vi "calc target data.vi"(8 "error in (no error)":errorcluster) -> (0 "error out":errorcluster, 1 "D":dbl=167.6323165634755, 2 "TARGET (XY)":T1 {"Y" format="%.4g"; "X" format="%.4g"}, 3 "steer (deg)":dbl=-10.0)   [LabVIEW 2023]
uses:
  ctrl defs/ctrl XY coord.ctl
  Global odometry.vi
  Global INIT.vi
  <vilib>/Rock Robotics/WPI/ThirdParty/JAS_Junk/TrajLib/Trajectory_Library.lvlib
panel:
  out "Inches":dbl
  out "DistanceToTarget_Meters":dbl
  in  "TEST":bool
  out "Dx":dbl=-165.57299375482046
  out "Dy":dbl=26.19498607564902
  out "ty":dbl=-15.0
  out "tx":dbl=-10.0
  out "tx angle error":dbl
  out "angle":dbl=22.0
  out "Z":dbl=22.0
  out "Y":dbl=-3.0
  out "X":dbl
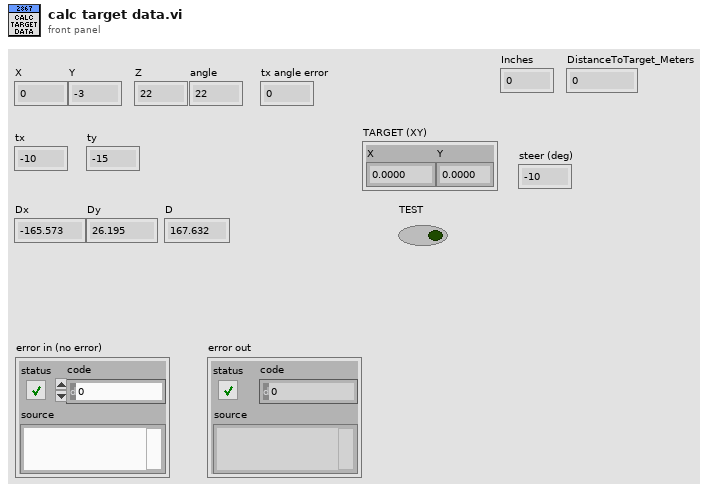
[diagram p1: front panel]
types:
  T1 = typedef "ctrl XY coord.ctl" = cluster{"X":dbl, "Y":dbl}
  T2 = typedef "ctrl LIMELIGHT initialize.ctl" = cluster{"Installed?":bool, "pose":cluster{"X":dbl, "Y":dbl, "Z":dbl, "angle to horizon":dbl, "tx angle offset":dbl}}
  T3 = typedef "ctrl LimeLight target.ctl" = cluster{"tv":u8, "tx":dbl, "ty":dbl, "ta":dbl}
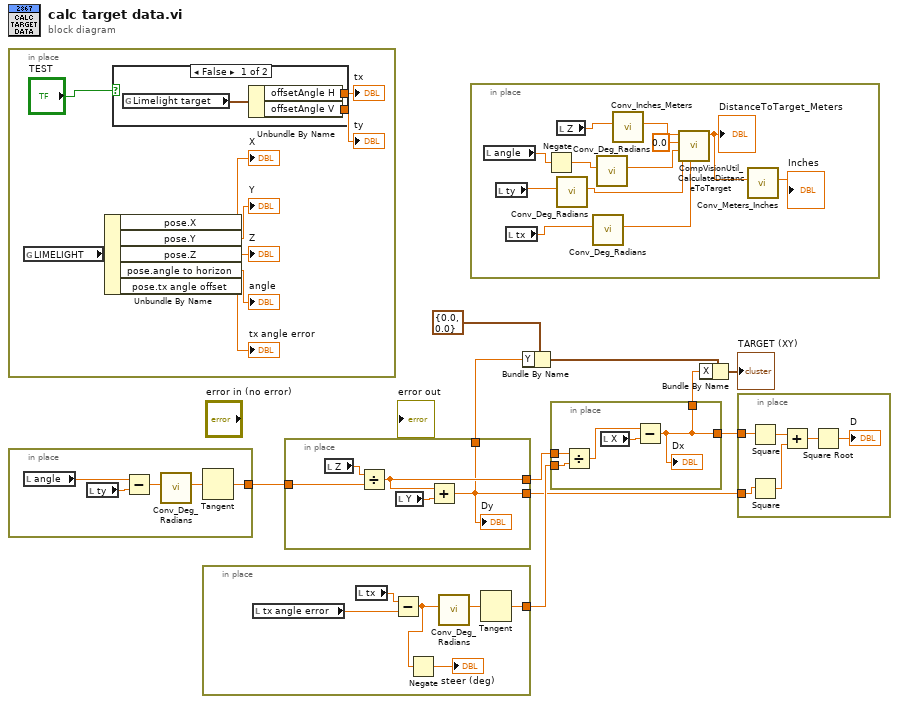
[diagram p0: block diagram]
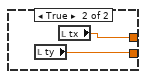
[diagram p2: hidden frame]
diagram:
  n1 = in-place {
    n2 = global read "Global INIT.vi" "LIMELIGHT"() -> (w19:T2)
    n3 = Unbundle By Name(w19) -> ("pose.X"=→"X":dbl, "pose.Y"=→"Y":dbl, "pose.Z"=→"Z":dbl, "pose.angle to horizon"=→"angle":dbl, "pose.tx angle offset"=→"tx angle error":dbl)
    n4 = case shown="False" "TEST" {
      tunnel: [w21 w24] -> w13
      tunnel: [w20 w23] -> w12
      frame False {
        n5 = global read "Global odometry.vi" "Limelight target"() -> (w22:T3)
        n6 = Unbundle By Name(w22) -> ("offsetAngle H"=w21:dbl, "offsetAngle V"=w20:dbl)
      }
      frame True {
        n7 = local read "ty"() -> (w23:dbl)
        n8 = local read "tx"() -> (w24:dbl)
      }
    }
    "tx" <- w13
    "ty" <- w12
  }
  n9 = in-place {
    in-place-border: [w25] -> w10
    n10 = local read "angle"() -> (w29:dbl)
    n11 = local read "ty"() -> (w28:dbl)
    n12 = Subtract(x=w29, y=w28) -> (x-y=w27:dbl)
    n13 = call <vilib>:"Conv_Deg_Radians.vi"("Degress"=w27) -> ("Radians"=w26:dbl)  [unwired: 10 in]
    n14 = Tangent(1:w26) -> (0:w25:dbl)
  }
  n15 = in-place {
    in-place-border: [w32] -> w8
    n16 = local read "tx angle error"() -> (w33:dbl)
    n17 = local read "tx"() -> (w34:dbl)
    n18 = Subtract(x=w34, y=w33) -> (x-y=w30:dbl)
    n19 = Negate(x=w30) -> (-x=→"steer (deg)":dbl)
    n20 = call <vilib>:"Conv_Deg_Radians.vi"("Degress"=w30) -> ("Radians"=w35:dbl)  [unwired: 10 in]
    n21 = Tangent(1:w35) -> (0:w32:dbl)
  }
  n22 = in-place {
    in-place-border: w10 -> [w39]
    in-place-border: [w37] -> w9
    in-place-border: [w36] -> w7
    in-place-border: [w36] -> w4
    n23 = local read "Z"() -> (w40:dbl)
    n24 = Divide(x=w40, y=w39) -> (x/y=w37:dbl)
    n25 = local read "Y"() -> (w38:dbl)
    n26 = Add(x=w37, y=w38) -> (x+y=w36:dbl)
    "Dy" <- w36
  }
  n27 = in-place {
    n28 = local read "angle"() -> (w47:dbl)
    n29 = local read "ty"() -> (w46:dbl)
    n30 = local read "tx"() -> (w44:dbl)
    n31 = Negate(x=w47) -> (-x=w48:dbl)
    n32 = local read "Z"() -> (w52:dbl)
    n33 = call <vilib>:"Conv_Deg_Radians.vi"("Degress"=w46) -> ("Radians"=w45:dbl)  [unwired: 10 in]
    n34 = call <vilib>:"Conv_Deg_Radians.vi"("Degress"=w44) -> ("Radians"=w43:dbl)  [unwired: 10 in]
    n35 = call <vilib>:"Conv_Deg_Radians.vi"("Degress"=w48) -> ("Radians"=w49:dbl)  [unwired: 10 in]
    n36 = call <vilib>:"Conv_Inches_Meters.vi"("INCH"=w52) -> ("Meters"=w51:dbl)  [unwired: 10 in]
    n37 = call <vilib>:"CompVisionUtil_CalculateDistanceToTarget.vi"("TargetYawRadians"=w43, "targetPitch_Radians"=w45, "cameraPitch_Radians"=w49, "targetHeight_Meters"=0.0, "cameraHeight_Meters"=w51) -> ("DistanceToTarget_Meters"=w42:dbl)  [unwired: 6 in]
    "DistanceToTarget_Meters" <- w42
    n38 = call <vilib>:"Conv_Meters_Inches.vi"("Meters"=w42) -> ("Inches"=→"Inches":dbl)  [unwired: 10 in]
  }
  n39 = Bundle By Name(cluster=T1 {"X"=0.0, "Y"=0.0} ("pivot center"), "Y"=w4) -> (w3:T1)
  n40 = in-place {
    in-place-border: w9 -> [w57]
    in-place-border: w8 -> [w56]
    in-place-border: [w53] -> w6
    in-place-border: [w53] -> w2
    n41 = Divide(x=w57, y=w56) -> (x/y=w55:dbl)
    n42 = local read "X"() -> (w54:dbl)
    n43 = Subtract(x=w55, y=w54) -> (x-y=w53:dbl)
    "Dx" <- w53
  }
  n44 = Bundle By Name(cluster=w3, "X"=w2) -> (→"TARGET (XY)":T1)
  n45 = in-place {
    in-place-border: w7 -> [w63]
    in-place-border: w6 -> [w62]
    n46 = Square(x=w62) -> (x^2=w61:dbl)
    n47 = Square(x=w63) -> (x^2=w60:dbl)
    n48 = Add(x=w61, y=w60) -> (x+y=w59:dbl)
    n49 = Square Root(x=w59) -> (sqrt(x)=→"D":dbl)
  }
